vi "ruby_pression.vi"() -> ()   [LabVIEW 2018]
panel:
  in  "Lambda, P0":dbl=694.24
  out "Pressure /GPa":dbl format="%.2f"
  in  "R1 peak":dbl(slide)=694.24 min=694.2 max=710.0 step=0.01 scale=694.24..710.0
  in  "stop":bool
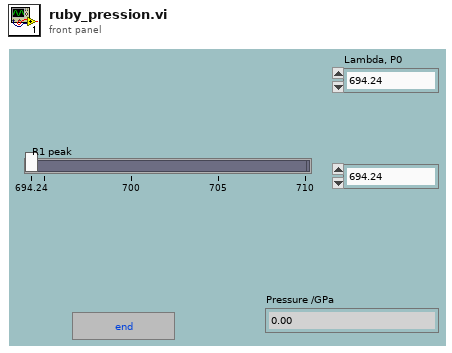
[diagram p1: front panel]
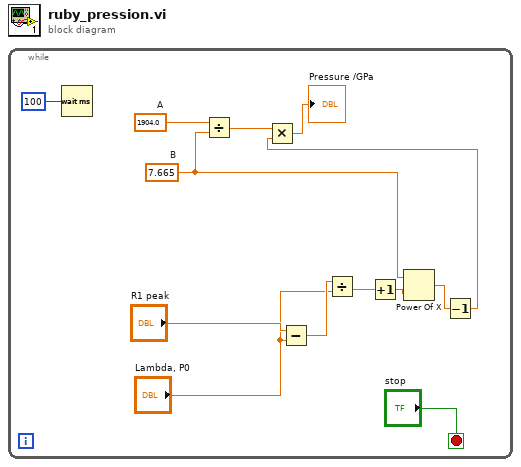
[diagram p0: block diagram]
diagram:
  n1 = while {
    stop <- "stop" stop-if-true
    w5 = 7.665  # B
    w12 = 1904.0  # A
    n2 = Wait (ms)(milliseconds to wait=u32 100 ("attente (ms)")) -> ()  [unwired: 1 out]
    n3 = Divide(x=w12, y=w5) -> (x/y=w11:dbl)
    n4 = Subtract(x="R1 peak", y="Lambda, P0") -> (x-y=w9:dbl)
    n5 = Divide(x=w9, y="Lambda, P0") -> (x/y=w7:dbl)
    n6 = Increment(x=w7) -> (x+1=w6:dbl)
    n7 = Power Of X(1:w6, 2:w5) -> (0:w4:dbl)
    n8 = Decrement(x=w4) -> (x-1=w3:dbl)
    n9 = Multiply(x=w11, y=w3) -> (x*y=→"Pressure /GPa":dbl)
  }
